vi "HFRR ADV v019 new software.vi"() -> ()   [LabVIEW 2025] (continued)
                        n2544 = disable-structure shown="Disabled" {
                          frame Disabled {
                            n2545 = local read "EVENT LOG"() -> (w3561:string)
                            n2546 = call "Event Log.vi"("Content"="Test Parameter", "EVENT LOG"=w3561) -> ("EVENT LOG"=w3560:string)  [unwired: 8 in, 1 out]
                            n2547 = local write "EVENT LOG"(w3560) -> ()
                          }
                          frame Enabled {
                          }
                        }
                      }
                      frame #20 {
                        n2548 = Wait (ms)(milliseconds to wait=u32 50) -> ()  [unwired: 1 out]
                      }
                      frame #21 {
                        n2549 = local read "Set Hz"() -> (w3565:dbl)
                        n2550 = Number To Fractional String(number=w3565, precision (6)=i16 2) -> (F-format string=w3564:string)  [unwired: 2 in]
                        n2551 = Concatenate Strings("Set Frequency [Hz] :" ("Content"), w3564) -> (w3567:string)
                        n2552 = local read "EVENT LOG"() -> (w3569:string)
                        n2553 = call "Event Log.vi"("Content"=w3567, "EVENT LOG"=w3569) -> ("EVENT LOG"=w3568:string)  [unwired: 8 in, 1 out]
                        n2554 = local write "EVENT LOG"(w3568) -> ()
                      }
                      frame #22 {
                        n2555 = Wait (ms)(milliseconds to wait=u32 50) -> ()  [unwired: 1 out]
                      }
                      frame #23 {
                        n2556 = local read "NORMAL LOAD"() -> (w3572:dbl)
                        n2557 = Number To Fractional String(number=w3572, precision (6)=i16 2) -> (F-format string=w3573:string)  [unwired: 2 in]
                        n2558 = Concatenate Strings("Applied Load [grams] :" ("Content"), w3573) -> (w3575:string)
                        n2559 = local read "EVENT LOG"() -> (w3577:string)
                        n2560 = call "Event Log.vi"("Content"=w3575, "EVENT LOG"=w3577) -> ("EVENT LOG"=w3576:string)  [unwired: 8 in, 1 out]
                        n2561 = local write "EVENT LOG"(w3576) -> ()
                      }
                      frame #24 {
                        n2562 = Wait (ms)(milliseconds to wait=u32 50) -> ()  [unwired: 1 out]
                      }
                      frame #25 {
                        n2563 = local read "Set Strk"() -> (w3580:dbl)
                        n2564 = Number To Fractional String(number=w3580, precision (6)=i16 2) -> (F-format string=w3581:string)  [unwired: 2 in]
                        n2565 = Concatenate Strings("Set Stroke [mm] :" ("Content"), w3581) -> (w3583:string)
                        n2566 = local read "EVENT LOG"() -> (w3585:string)
                        n2567 = call "Event Log.vi"("Content"=w3583, "EVENT LOG"=w3585) -> ("EVENT LOG"=w3584:string)  [unwired: 8 in, 1 out]
                        n2568 = local write "EVENT LOG"(w3584) -> ()
                      }
                      frame #26 {
                        n2569 = Wait (ms)(milliseconds to wait=u32 50) -> ()  [unwired: 1 out]
                      }
                      frame #27 {
                        n2570 = local read "Set Temp"() -> (w3588:dbl)
                        n2571 = Number To Fractional String(number=w3588, precision (6)=i16 2) -> (F-format string=w3589:string)  [unwired: 2 in]
                        n2572 = Concatenate Strings("Set Temperature [deg C] :" ("Content"), w3589) -> (w3591:string)
                        n2573 = local read "EVENT LOG"() -> (w3593:string)
                        n2574 = call "Event Log.vi"("Content"=w3591, "EVENT LOG"=w3593) -> ("EVENT LOG"=w3592:string)  [unwired: 8 in, 1 out]
                        n2575 = local write "EVENT LOG"(w3592) -> ()
                      }
                      frame #28 {
                        n2576 = Wait (ms)(milliseconds to wait=u32 50) -> ()  [unwired: 1 out]
                      }
                      frame #29 {
                        n2577 = local read "Set Rh"() -> (w3596:dbl)
                        n2578 = Number To Fractional String(number=w3596, precision (6)=i16 2) -> (F-format string=w3597:string)  [unwired: 2 in]
                        n2579 = Concatenate Strings("Set Humidity [%RH] :" ("Content"), w3597) -> (w3599:string)
                        n2580 = local read "EVENT LOG"() -> (w3601:string)
                        n2581 = call "Event Log.vi"("Content"=w3599, "EVENT LOG"=w3601) -> ("EVENT LOG"=w3600:string)  [unwired: 8 in, 1 out]
                        n2582 = local write "EVENT LOG"(w3600) -> ()
                      }
                      frame #30 {
                        n2583 = Wait (ms)(milliseconds to wait=u32 50) -> ()  [unwired: 1 out]
                      }
                      frame #31 {
                        n2584 = local read "test time"() -> (w3604:dbl)
                        n2585 = Number To Fractional String(number=w3604, precision (6)=i16 1) -> (F-format string=w3605:string)  [unwired: 2 in]
                        n2586 = Concatenate Strings("Test Duration [mins] :" ("Content"), w3605) -> (w3607:string)
                        n2587 = local read "EVENT LOG"() -> (w3609:string)
                        n2588 = call "Event Log.vi"("Content"=w3607, "EVENT LOG"=w3609) -> ("EVENT LOG"=w3608:string)  [unwired: 8 in, 1 out]
                        n2589 = local write "EVENT LOG"(w3608) -> ()
                      }
                      frame #32 {
                        w3610 = dbl[] [] ("History Data")
                        w3611 = cluster{"y":dbl, dbl, "y":dbl}[] [] ("History Data")
                        w3612 = FALSE ("Visible")
                        n2590 = property on="Stroke ( mm )" class="WFChart (strict)"("History Data"=w3611) -> ()  [unwired: 2 in, 2 out]
                        n2591 = property on="Humidity ( %RH )" class="WFChart (strict)"("History Data"=w3610) -> ()  [unwired: 2 in, 2 out]
                        n2592 = property on="Temperature ( Deg C )" class="WFChart (strict)"("History Data"=w3610) -> ()  [unwired: 2 in, 2 out]
                        n2593 = property on="Electrical Contact Resistance ( % )" class="WFChart (strict)"("History Data"=w3610) -> ()  [unwired: 2 in, 2 out]
                        n2594 = property on="Coefficient of Friction" class="WFChart (strict)"("History Data"=w3610) -> ()  [unwired: 2 in, 2 out]
                        n2595 = property on="Frictional Force ( N )" class="WFChart (strict)"("History Data"=w3610) -> ()  [unwired: 2 in, 2 out]
                        n2596 = property on="Coefficient of Friction" class="WFChart (strict)"("History Data"=w3610) -> ()  [unwired: 2 in, 2 out]
                        n2597 = property on="Frictional Force ( N )" class="WFChart (strict)"("History Data"=w3610) -> ()  [unwired: 2 in, 2 out]
                        n2598 = property on="Electrical Contact Resistance ( % )" class="WFChart (strict)"("History Data"=w3610) -> ()  [unwired: 2 in, 2 out]
                        n2599 = property on="Humidity ( %RH )" class="WFChart (strict)"("History Data"=w3610) -> ()  [unwired: 2 in, 2 out]
                        n2600 = property on="Stroke ( mm )" class="WFChart (strict)"("History Data"=w3611) -> ()  [unwired: 2 in, 2 out]
                        n2601 = property on="Temperature ( Deg C )" class="WFChart (strict)"("History Data"=w3610) -> ()  [unwired: 2 in, 2 out]
                        n2602 = property on="Service Password Log" class="Str"("Visible"=w3612) -> ()  [unwired: 2 in, 2 out]
                        n2603 = property on="Password 3" class="Clust (strict)"("Visible"=w3612) -> ()  [unwired: 2 in, 2 out]
                      }
                    }
                    "TEST FILE NAM,E SAVED" <- TRUE ("TEST FILE NAM,E SAVED")
                  }
                }
              }
            }
          }
        }
        n2604 = case shown="True" w2909 {
          frame False {
            n2605 = local write "tfalg"(0.0 ("tfalg")) -> ()
          }
          frame True {
            n2606 = local read "tfalg"() -> (w3054:dbl)
            n2607 = Equal?(x=w3054, y=0.0) -> (x = y?=w3055:bool)
            n2608 = case shown="True" w3055 {
              frame False {
              }
              frame True {
                n2609 = local read "Total No. of Tests"() -> (w3058:dbl)
                n2610 = local write "tfalg"(1.0 ("tfalg")) -> ()
                n2611 = local write "acq 2"(FALSE ("acq 2")) -> ()
                n2612 = Wait (ms)(milliseconds to wait=u32 200) -> ()  [unwired: 1 out]
                n2613 = Increment(x=w3058) -> (x+1=w3057:dbl)
                n2614 = local write "Total No. of Tests"(w3057) -> ()
              }
            }
          }
        }
        n2615 = local write "Test \nStatus"(w2915) -> ()
        n2616 = local write "Save"(w2915) -> ()
        n2617 = local read "Main Tab"() -> (w2872:T2)
        n2618 = case shown="True" w2896 {
          tunnel: [FALSE ("RUN") TRUE ("RUN")] -> w2895
          tunnel: [_ 1] -> w2888
          frame False {
          }
          frame True {
          }
        }
        n2619 = In Range and Coerce(upper limit=w2903, x=w2876, lower limit=w2902) -> (In Range?=w2894:bool)  [unwired: 1 out]
        n2620 = In Range and Coerce(upper limit=w2900, x=w2875, lower limit=w2901) -> (In Range?=w2892:bool)  [unwired: 1 out]
        n2621 = case shown="True" w2908 {
          frame False {
            n2622 = local read "Rt 3"() -> (w3036:bool)
            n2623 = case shown="True" w3036 {
              frame False {
              }
              frame True {
                n2624 = local write "Rt 3"(FALSE ("Rt 3")) -> ()
                n2625 = local write "Json End Flg"(TRUE ("Upld AR 2")) -> ()
              }
            }
            "Rt" <- TRUE ("Rt")
            "Rt 2" <- FALSE ("Rt")
          }
          frame True {
            n2626 = local read "Rt"() -> (w3043:bool)
            n2627 = local write "Rt 2"(TRUE ("Rt 2")) -> ()
            n2628 = case shown="True" w3043 {
              frame False {
              }
              frame True {
                w3044 = TRUE ("Upld AR 2")
                n2629 = local write "Rt"(FALSE ("Rt")) -> ()
                n2630 = local write "Upld AR"(w3044) -> ()
                n2631 = local write "Json St Flg"(w3044) -> ()
              }
            }
            "Rt 3" <- TRUE ("Rt 3")
          }
        }
        n2632 = case shown="True" w2894 {
          tunnel: [FALSE ("RUN") TRUE ("RUN")] -> w2893
          tunnel: [_ 2] -> w2887
          frame False {
          }
          frame True {
          }
        }
        n2633 = case shown="True" w2892 {
          tunnel: [FALSE ("RUN") TRUE ("RUN")] -> w2891
          tunnel: [_ 3] -> w2886
          frame False {
          }
          frame True {
          }
        }
        n2634 = case shown="\"Acquire\"" w2872 {
          tunnel: w2874 -> [_ w3105]
          frame Default {
            w3104 = 0.0 ("output")
            n2635 = local write "PID-out"(w3104) -> ()
            n2636 = local write "Frequency ( Hz )"(w3104) -> ()
          }
          frame "Acquire" {
            n2637 = stacked-sequence {
              frame #0 {
                n2638 = local read "Auto Start Test"() -> (w3107:bool)
                n2639 = case shown="True" w3107 {
                  tunnel: "RUN" -> [w3128 w3131]
                  tunnel: [w3128 w3130] -> w3108
                  frame False {
                  }
                  frame True {
                    n2640 = local read "Auto Start Temp"() -> (w3129:bool)
                    n2641 = Or(x=w3131, y=w3129) -> (x .or. y?=w3130:bool)
                  }
                }
                n2642 = local read "clk"() -> (w3127:dbl)
                n2643 = local read "Save"() -> (w3123:bool)
                n2644 = Equal?(x=w3127, y=0.0) -> (x = y?=w3124:bool)
                n2645 = And(x=w3124, y=w3123) -> (x .and. y?=w3125:bool)
                n2646 = Not(x="Engage") -> (.not. x?=w3114:bool)
                n2647 = case shown="False" w3108 {
                  tunnel: [0.0 w3154] -> w3110
                  frame False {
                    (unwired) TRUE ("Visible")
                    n2648 = local read "Auto Start Test"() -> (w3135:bool)
                    n2649 = local write "Start Time"(TRUE ("Start Time")) -> ()
                    n2650 = property on="Stroke 2" class="DigNum (strict)"("Visible"=FALSE) -> ()  [unwired: 2 in, 2 out]
                    n2651 = case shown="False" w3135 {
                      frame False {
                        n2652 = property on="Heater Button" class="Bool (strict)"("DisabledEnum"=T19."Enabled" ("Disabled")) -> ()  [unwired: 2 in, 2 out]
                        n2653 = property on="Humidity" class="Bool (strict)"("DisabledEnum"=T19."Enabled" ("Disabled")) -> ()  [unwired: 2 in, 2 out]
                      }
                      frame True {
                      }
                    }
                    n2654 = case shown="False" "TestCompFlg" {
                      frame False {
                        n2655 = local read "StartFlg"() -> (w3143:bool)
                        n2656 = case shown="True" w3143 {
                          frame False {
                          }
                          frame True {
                            n2657 = stacked-sequence {
                              frame #0 {
                                n2658 = local read "EVENT LOG"() -> (w3147:string)
                                n2659 = call "Event Log.vi"("Content"="Test was interrupted", "EVENT LOG"=w3147) -> ("EVENT LOG"=w3148:string)  [unwired: 8 in, 1 out]
                                n2660 = local write "EVENT LOG"(w3148) -> ()
                                n2661 = property on="RUN" class="Bool (strict)"("Visible"=TRUE) -> ()  [unwired: 2 in, 2 out]
                                n2662 = property on="Auto Start Test" class="Bool (strict)"("Visible"=TRUE) -> ()  [unwired: 2 in, 2 out]
                              }
                              frame #1 {
                                w3150 = FALSE ("StartFlg")
                                n2663 = property on="Heater Button" class="Bool (strict)"("Val(Sgnl)"=FALSE ("Value (Signaling)")) -> ()  [unwired: 2 in, 2 out]
                                n2664 = local write "Heater Button"(w3150) -> ()
                                n2665 = local write "StartFlg"(w3150) -> ()
                                n2666 = local write "Humidity"(w3150) -> ()
                              }
                              frame #2 {
                                n2667 = local write "Command"("VC;0" ("Command")) -> ()
                              }
                              frame #3 {
                                n2668 = Wait (ms)(milliseconds to wait=u32 1500) -> ()  [unwired: 1 out]
                              }
                              frame #4 {
                                n2669 = local write "Command"("HE;0" ("Command")) -> ()
                              }
                            }
                          }
                        }
                      }
                      frame True {
                      }
                    }
                    n2670 = local write "String 14"("Test will autostart once parameters reach the set value." ("String 14")) -> ()
                  }
                  frame True {
                    (unwired) FALSE ("Visible")
                    n2671 = property on="Stroke 2" class="DigNum (strict)"("Visible"=TRUE) -> ()  [unwired: 2 in, 2 out]
                    n2672 = property on="STOP 2" class="Bool (strict)"("Disabled"=u8 2) -> ()  [unwired: 2 in, 2 out]
                    n2673 = local write "String 14"(" Running....." ("String 14")) -> ()
                    n2674 = property on="Heater Button" class="Bool (strict)"("DisabledEnum"=T19."Disabled and Grayed Out" ("Disabled")) -> ()  [unwired: 2 in, 2 out]
                    n2675 = property on="Humidity" class="Bool (strict)"("DisabledEnum"=T19."Disabled and Grayed Out" ("Disabled")) -> ()  [unwired: 2 in, 2 out]
                    n2676 = case shown="True" "Start Time" {
                      selector: "Start Time" -> [_ w3173]
                      frame False {
                      }
                      frame True {
                        n2677 = Not(x=w3173) -> (.not. x?=w3172:bool)
                        n2678 = local write "Start Time"(w3172) -> ()
                        n2679 = local read "EVENT LOG"() -> (w3174:string)
                        n2680 = call "Event Log.vi"("Content"="Test in progress", "EVENT LOG"=w3174) -> ("EVENT LOG"=w3176:string)  [unwired: 8 in, 1 out]
                        n2681 = local write "EVENT LOG"(w3176) -> ()
                      }
                    }
                    n2682 = disable-structure shown="Enabled" {
                      disable-tunnel: [w3165 w3171] -> w3154
                      frame Disabled {
                        n2683 = local read "Set Hz"() -> (w3168:dbl)
                        n2684 = call <vilib>:"Uniform White Noise Waveform.vi"() -> ("signal out"=w3167:waveform(dbl))  [unwired: 10 in, 1 out]
                        n2685 = Random Number (0-1)() -> (number: 0 to 1=w3164:dbl)
                        n2686 = Add(x=w3168, y=w3167) -> (x+y=w3166:waveform(dbl))
                        n2687 = Multiply(x=ext 0.01 ("y"), y=w3164) -> (x*y=w3162:ext)
                        n2688 = Multiply(x=w3166, y=w3162) -> (x*y=w3165:waveform(ext))
                      }
                      frame Enabled {
                        n2689 = call-poly <vilib>:"Random Number (Range).vi"("lower bound (0)"=49.89, "upper bound (100)"=50.8) -> ("number"=w3171:dbl)  [unwired: 9 in]
                      }
                    }
                    "StartFlg" <- TRUE ("StartFlg")
                  }
                }
                n2690 = case shown="True" w3125 {
                  frame False {
                  }
                  frame True {
                    n2691 = local write "clk"(10.0 ("clk")) -> ()
                    n2692 = Get Date/Time In Seconds() -> (seconds since 1Jan1904=w3179:timestamp)
                    n2693 = To Double Precision Float(number=w3179) -> (double precision float=w3177:dbl)
                    n2694 = local write "acq timer"(w3177) -> ()
                    n2695 = local write "act save time"(w3177) -> ()
                  }
                }
                n2696 = call "Elapsed Time"("Time Target (s)"="Countdown", "Reset"=w3114) -> ("Elapsed Time (s)"=w3119:dbl, "Time has Elapsed"=w3117:bool)  [unwired: 10 in, 6 out]
                "Countdown 2" <- w3119
                n2697 = Subtract(x=w3119, y=2.0) -> (x-y=w3122:dbl)
                n2698 = Less?(x=w3122, y="Countdown") -> (x < y?=w3120:bool)
                n2699 = And(x=w3120, y=w3117) -> (x .and. y?=w3116:bool)
                n2700 = case shown="True" w3116 {
                  frame False {
                  }
                  frame True {
                    (unwired) dbl[] [] ("History Data")
                    n2701 = local write "Engage"(FALSE ("Engage")) -> ()
                    n2702 = local write "RUN"(TRUE ("RUN")) -> ()
                    n2703 = local read "Humidity ( %RH )"() -> (→"Rh Before":dbl)
                  }
                }
                n2704 = local read "Test \nStatus"() -> (w3112:bool)
                n2705 = Select(t=w3110, s=w3112, f=0.0) -> (s? t:f=w3111:dbl)
                n2706 = local write "Frequency ( Hz )"(w3111) -> ()
              }
              frame #1 {
                w3202 = 1000000.0 ("x")
                # "HC;1/0\nST;VALUE"
                # "Elapsed time\ncof\nstroke\nAir temp\nTemp\nHumidity"
                # "acq timer\n\nact save time"
                # "convert to microseconds"
                n2707 = local read "COUNT"() -> (w3185:i32)
                n2708 = local read "Rate"() -> (w3198:dbl)
                n2709 = Divide(x=w3202, y=w3198) -> (x/y=w3203:dbl)
                n2710 = Greater Or Equal?(x=w3185, y=250) -> (x >= y?=w3184:bool)
                n2711 = Get Date/Time In Seconds() -> (seconds since 1Jan1904=w3205:timestamp)
                n2712 = case shown="True" w3184 {
                  frame False {
                    n2713 = local read "COUNT"() -> (w3206:i32)
                    n2714 = Increment(x=w3206) -> (x+1=w3207:i32)
                    n2715 = local write "COUNT"(w3207) -> ()
                  }
                  frame True {
                    n2716 = local write "COUNT"(0 ("COUNT")) -> ()
                  }
                }
                n2717 = local read "Samplingtime 2"() -> (w3183:dbl)
                n2718 = local read "act save time"() -> (w3200:dbl)
                n2719 = Divide(x=w3203, y=w3202) -> (x/y=w3201:dbl)
                n2720 = To Double Precision Float(number=w3205) -> (double precision float=w3194:dbl)
                n2721 = Add(x=w3200, y=w3183) -> (x+y=w3199:dbl)
                n2722 = local read "acq timer"() -> (w3204:dbl)
                n2723 = local read "COUNT"() -> (w3187:i32)
                n2724 = Greater Or Equal?(x=w3194, y=w3199) -> (x >= y?=w3182:bool)
                n2725 = Multiply(x=w3201, y=w3187) -> (x*y=w3193:dbl)
                n2726 = Subtract(x=w3194, y=w3204) -> (x-y=w3196:dbl)
                n2727 = local read "Save"() -> (w3197:bool)
                n2728 = Add(x=w3196, y=w3193) -> (x+y=w3180:dbl)
                "Elapsed time 3" <- w3180
                n2729 = And(x=w3182, y=w3197) -> (x .and. y?=w3195:bool)
                n2730 = Divide(x=w3180, y=60.0) -> (x/y=w3191:dbl)
                n2731 = local read "Test \nStatus"() -> (w3181:bool)
                n2732 = local read "clk"() -> (w3188:dbl)
                n2733 = Equal?(x=w3188, y=10.0) -> (x = y?=w3190:bool)
                n2734 = case shown="True" w3195 {
                  tunnel: w3194 -> [_ w3318]
                  tunnel: [FALSE ("Boolean 2") TRUE ("Boolean 2")] -> _
                  frame False {
                  }
                  frame True {
                    w3272 = ";" ("Substring")
                    # "Pid out/\nFreq response value"
                    n2735 = local write "act save time"(w3318) -> ()
                    n2736 = local read "FILE"() -> (w3266:string)
                    n2737 = call "file check.vi"("file name in"=w3266) -> ("error out"=w3269:errorcluster, "file name out"=w3264:string)  [unwired: 9 in]
                    n2738 = local read "LVDT STROKE"() -> (w3261:dbl)
                    n2739 = local read "Add up Stroke"() -> (w3259:dbl)
                    n2740 = call "FILE PATH CREATION.vi"("error in"=w3269, "FILE NAME :"=w3264) -> ("FILE OUT"=w3267:path)  [unwired: 8 in, 1 out]
                    n2741 = Concatenate Strings(w3264, ".dgf" ("Substring")) -> (w3268:string)
                    n2742 = Subtract(x=w3261, y=w3259) -> (x-y=w3260:dbl)
                    n2743 = Absolute Value(x=w3260) -> (abs(x)=w3258:dbl)
                    n2744 = local read "FF 2"() -> (→"Frictional Force ( N )" →"Frictional Force ( N )":dbl)
                    n2745 = Build Path(base path=w3267, name or relative path=w3268) -> (appended path=w3263:path)
                    n2746 = local read "COF 2"() -> (w3277:dbl)
                    "cof" <- w3277
                    "Coefficient of Friction" <- w3277
                    "COF 4" <- w3277
                    "Coefficient of Friction" <- w3277
                    n2747 = local read "TEMP"() -> (w3280:dbl)
                    "Temp" <- w3280
                    "Temperature ( Deg C )" <- w3280
                    n2748 = local read "Humidity ( %RH )"() -> (w3279:dbl)
                    "Humidity ( %RH )" <- w3279
                    "Humidity ( %RH )" <- w3279
                    n2749 = local read "Frequency ( Hz )"() -> (w3286:dbl)
                    n2750 = call <vilib>:"Mean PtByPt.vi"("x"=w3258, "sample length"="STROKE FILTER") -> ("mean"=w3257:dbl)  [unwired: 2 in, 1 out]
                    n2751 = local read "Elapsed time"() -> (w3311:dbl)
                    n2752 = local read "AIR TEMP"() -> (w3284:dbl)
                    n2753 = local read "PID-out"() -> (w3289:dbl)
                    n2754 = local write "Temperature ( Deg C )"(w3280) -> ()
                    n2755 = Number To Fractional String(number=w3257, width (-)=i16 9 ("precision (6)"), precision (6)=i16 6) -> (F-format string=w3304:string)  [unwired: 1 in]
                    n2756 = Number To Fractional String(number=w3284, width (-)=i16 9 ("precision (6)"), precision (6)=i16 3) -> (F-format string=w3303:string)  [unwired: 1 in]
                    n2757 = Number To Fractional String(number=w3280, width (-)=i16 9 ("precision (6)"), precision (6)=i16 3) -> (F-format string=w3300:string)  [unwired: 1 in]
                    n2758 = Number To Fractional String(number=w3279, width (-)=i16 9 ("precision (6)"), precision (6)=i16 3) -> (F-format string=w3297:string)  [unwired: 1 in]
                    n2759 = Number To Fractional String(number=0.0, width (-)=i16 9 ("precision (6)"), precision (6)=i16 3) -> (F-format string=w3294:string)  [unwired: 1 in]
                    n2760 = Number To Fractional String(number=w3289, width (-)=i16 9 ("precision (6)"), precision (6)=i16 3) -> (F-format string=w3290:string)  [unwired: 1 in]
                    n2761 = Number To Fractional String(number=w3286, width (-)=i16 9 ("precision (6)"), precision (6)=i16 3) -> (F-format string=w3285:string)  [unwired: 1 in]
                    n2762 = Number To Fractional String(number=w3277, width (-)=i16 9 ("precision (6)"), precision (6)=i16 6) -> (F-format string=w3312:string)  [unwired: 1 in]
                    n2763 = Number To Fractional String(number=w3311, width (-)=i16 14 ("precision (6)"), precision (6)=i16 3) -> (F-format string=w3313:string)  [unwired: 1 in]
                    n2764 = Bundle("y"=1.02, "mean"=w3257, "y"=0.98) -> (w3278:cluster{"y":dbl, "mean":dbl, "y":dbl})  [unwired: 1 in]
                    n2765 = Number To Fractional String(number="Ambient Humidity :", width (-)=i16 9 ("precision (6)"), precision (6)=i16 6) -> (F-format string=w3270:string)  [unwired: 1 in]
                    n2766 = local read "RUN"() -> (w3276:bool)
                    n2767 = case shown="True" w3276 {
                      tunnel: w3278 -> [_ w3323]
                      tunnel: w3257 -> [_ w3322]
                      tunnel: w3257 -> [_ w3320]
                      tunnel: w3257 -> [_ w3321]
                      frame False {
                      }
                      frame True {
                        "Stroke ( mm )" <- w3323
                        "Stroke ( mm )" <- w3323
                        "Stroke 4" <- w3322
                        "Stroke 3" <- w3320
                        "Stroke 2" <- w3321
                        "measured_stroke" <- w3320
                      }
                    }
                    n2768 = Concatenate Strings(w3313, w3272, w3312, w3272, w3304, w3272, w3303, w3272, w3300, w3272, w3297, w3272, w3294, w3272, w3290, w3272, w3285, w3272, w3270, "\r") -> (w3310:string)
                    n2769 = call <vilib>:"Write Characters To File.vi"("append to file? (new file:F)"=TRUE, "character string"=w3310, "file path (dialog if empty)"=w3263) -> ()  [unwired: 2 in, 1 out]
                    "refresh flag" <- TRUE ("refresh flag")
                  }
                }
                n2770 = case shown="True" w3181 {
                  tunnel: w3191 -> [_ w3217]
                  tunnel: w3196 -> [_ w3227]
                  tunnel: [0.0 w3223] -> _
                  tunnel: w3190 -> [_ w3222]
                  tunnel: [0.0 w3221] -> _
                  tunnel: w3180 -> [_ w3221]
                  tunnel: w3194 -> [w3210 _]
                  frame False {
                    n2771 = local write "acq timer"(w3210) -> ()
                    n2772 = local write "Test Duration Status"(0.0 ("Test Duration Status")) -> ()
                  }
                  frame True {
                    n2773 = local read "Set Hz"() -> (w3224:dbl)
                    n2774 = local write "Elapsed time"(w3217) -> ()
                    n2775 = local read "test time"() -> (w3216:dbl)
                    n2776 = Multiply(x=w3227, y=w3224) -> (x*y=w3226:dbl)
                    n2777 = case shown="False" w3222 {
                      tunnel: w3226 -> [w3228 _]
                      tunnel: [w3228 1.0] -> w3223
                      frame False {
                        n2778 = local write "Cycles elapsed"(w3228) -> ()
                      }
                      frame True {
                      }
                    }
                    n2779 = Greater?(x=w3217, y=w3216) -> (0:w3225:bool)
                    n2780 = Subtract(x=w3216, y=w3217) -> (x-y=w3215:dbl)
                    "time" <- w3215
                    n2781 = Multiply(x=w3215, y=60.0) -> (x*y=w3214:dbl)
                    n2782 = local write "Time Remaining"(w3214) -> ()
                    n2783 = local write "Remaining Time"(w3214) -> ()
                    n2784 = case shown="True" w3225 {
                      frame False {
                      }
                      frame True {
                        n2785 = stacked-sequence {
                          frame #0 {
                            w3233 = T19."Enabled" ("Disabled")
                            w3232 = FALSE ("TEST FILE NAM,E SAVED")
                            w3234 = "" ("FILE")
                            w3235 = TRUE ("Visible")
                            n2786 = local write "Humidity"(FALSE ("Humidity")) -> ()
                            n2787 = local write "RUN"(FALSE ("OK Button 2")) -> ()
                            n2788 = local write "Heater Button"(FALSE ("Heater Button")) -> ()
                            n2789 = local write "Auto Start Test"(FALSE ("Auto Start Test")) -> ()
                            n2790 = local write "TestCompFlg"(TRUE ("StpFlg")) -> ()
                            n2791 = local read "Humidity ( %RH )"() -> (→"Rh After":dbl)
                            n2792 = property on="STOP 2" class="Bool (strict)"("Disabled"=u8 0) -> ()  [unwired: 2 in, 2 out]
                            n2793 = local read "EVENT LOG"() -> (w3240:string)
                            n2794 = call "Event Log.vi"("Content"="Test Completed", "EVENT LOG"=w3240) -> ("EVENT LOG"=w3239:string)  [unwired: 8 in, 1 out]
                            n2795 = property on="RUN" class="Bool (strict)"("Visible"=w3235) -> ()  [unwired: 2 in, 2 out]
                            n2796 = property on="Auto Start Test" class="Bool (strict)"("Visible"=w3235) -> ()  [unwired: 2 in, 2 out]
                            n2797 = local write "Batch Ref Num :"(w3234) -> ()
                            n2798 = local write "FILE"(w3234) -> ()
                            n2799 = local write "EVENT LOG"(w3239) -> ()
                            n2800 = local write "TEST FILE NAM,E SAVED"(w3232) -> ()
                            n2801 = local write "Fuel Discription :"(w3234) -> ()
                            n2802 = local write "START TEMP"(w3232) -> ()
                            n2803 = local write "Remarks :"(w3234) -> ()
                            n2804 = local write "Main Dashboard Buttons"(T1."Imaging" ("Main Dashboard Buttons")) -> ()
                            n2805 = local write "Main Tab"(T2."Adv Scar" ("Main Tab")) -> ()
                            n2806 = property on="FRICVALZ 2" class="Bool (strict)"("DisabledEnum"=w3233) -> ()  [unwired: 2 in, 2 out]
                            n2807 = property on="FRICVALZ 3" class="Bool (strict)"("DisabledEnum"=w3233) -> ()  [unwired: 2 in, 2 out]
                            n2808 = property on="FRICVALZ 4" class="Bool (strict)"("DisabledEnum"=w3233) -> ()  [unwired: 2 in, 2 out]
                          }
                          frame #1 {
                            n2809 = Wait (ms)(milliseconds to wait=u32 1500) -> ()  [unwired: 1 out]
                          }
                          frame #2 {
                            n2810 = local write "Command"("VC;0") -> ()
                          }
                          frame #3 {
                            n2811 = Wait (ms)(milliseconds to wait=u32 1500) -> ()  [unwired: 1 out]
                          }
                          frame #4 {
                            n2812 = local write "Command"("VC;0") -> ()
                          }
                          frame #5 {
                            n2813 = Wait (ms)(milliseconds to wait=u32 1500) -> ()  [unwired: 1 out]
                          }
                          frame #6 {
                            n2814 = local write "Command"("ST;0") -> ()
                          }
                          frame #7 {
                            n2815 = local write "measured_stroke"(0.0 ("measured_stroke")) -> ()
                            n2816 = Wait (ms)(milliseconds to wait=u32 1500) -> ()  [unwired: 1 out]
                          }
                          frame #8 {
                            n2817 = local write "Command"("HE;0") -> ()
                          }
                        }
                      }
                    }
                    n2818 = Divide(x=w3217, y=w3216) -> (x/y=w3220:dbl)
                    n2819 = Multiply(x=w3220, y=100.0) -> (x*y=w3218:dbl)
                    n2820 = local write "Test Duration Status"(w3218) -> ()
                  }
                }
              }
              frame #2 {
                n2821 = case shown="True" "Heater Button" {
                  tunnel: [0.0 ("output") w3346] -> w3324
                  frame False {
                    w3327 = TRUE ("tmpchk")
                    n2822 = local read "TEMP"() -> (w3328:dbl)
                    n2823 = local write "Temp ini"(w3328) -> ()
                    n2824 = local write "Reset 4"(w3327) -> ()
                    n2825 = local write "tmpchk"(w3327) -> ()
                    n2826 = local write "reinit"(TRUE ("reinit")) -> ()
                    n2827 = local write "manual temp log"(TRUE ("manual temp log")) -> ()
                  }
                  frame True {
                    # "Logic to turn off\nthe heater when \ntemp is not rising.\nTime - 60 sec\nDelta t- 5°c"
                    n2828 = local read "Temp ini"() -> (w3335:dbl)
                    n2829 = local read "Auto Start Test"() -> (w3331:bool)
                    n2830 = Less?(x=w3335, y=53.0) -> (x < y?=w3333:bool)
                    n2831 = case shown="False" w3331 {
                      frame False {
                        n2832 = local read "Set Temp"() -> (w3355:dbl)
                        n2833 = local read "TEMP"() -> (w3354:dbl)
                        n2834 = Subtract(x=w3355, y=w3354) -> (x-y=w3353:dbl)
                        n2835 = Absolute Value(x=w3353) -> (abs(x)=w3352:dbl)
                        n2836 = Less?(x=w3352, y=0.5) -> (x < y?=w3350:bool)
                        n2837 = case shown="True" w3350 {
                          tunnel: "manual temp log" -> [_ w3356]
                          frame False {
                          }
                          frame True {
                            n2838 = case shown="True" w3356 {
                              selector: w3356 -> [_ w3357]
                              frame False {
                              }
                              frame True {
                                # "#Event log"
                                n2839 = Not(x=w3357) -> (.not. x?=w3358:bool)
                                n2840 = local write "manual temp log"(w3358) -> ()
                                n2841 = local read "EVENT LOG"() -> (w3361:string)
                                n2842 = call "Event Log.vi"("Content"="Target Temperature reached", "EVENT LOG"=w3361) -> ("EVENT LOG"=w3360:string)  [unwired: 8 in, 1 out]
                                n2843 = local write "EVENT LOG"(w3360) -> ()
                              }
                            }
                          }
                        }
                      }
                      frame True {
                        n2844 = local write "manual temp log"(TRUE ("manual temp log")) -> ()
                      }
                    }
                    n2845 = And(x="tmpchk", y=w3333) -> (x .and. y?=w3336:bool)
                    n2846 = case shown="True" w3336 {
                      frame False {
                      }
                      frame True {
                        n2847 = call "Elapsed Time8"("Time Target (s)"=300.0, "Reset"="Reset 4") -> ("Time has Elapsed"=w3363:bool)  [unwired: 10 in, 7 out]
                        n2848 = flat-sequence {
                          tunnel: w3363 -> [_]
                          frame #0 {
                            n2849 = local write "Reset 4"(FALSE ("Reset 4")) -> ()
                          }
                        }
                        n2850 = case shown="True" w3363 {
                          frame False {
                          }
                          frame True {
                            n2851 = local read "Temp ini"() -> (w3370:dbl)
                            n2852 = Add(x=w3370, y=5.0) -> (x+y=w3368:dbl)
                            n2853 = local read "TEMP"() -> (w3371:dbl)
                            n2854 = Greater?(x=w3371, y=w3368) -> (0:w3369:bool)
                            n2855 = case shown="False" w3369 {
                              frame False {
                                n2856 = local write "Heater Button"(FALSE ("Heater Button")) -> ()
                              }
                              frame True {
                                n2857 = local write "tmpchk"(FALSE ("tmpchk")) -> ()
                              }
                            }
                          }
                        }
                      }
                    }
                    n2858 = local read "Set Temp"() -> (w3344:dbl)
                    n2859 = local read "TEMP"() -> (w3338:dbl)
                    n2860 = call-poly <vilib>:"PID.vi"("reinitialize? (F)"="reinit", "dt (s)"=-1.0, "process variable"=w3338, "setpoint"=w3344) -> ("output"=w3341:dbl)  [unwired: 6 in, 1 out]
                    n2861 = Subtract(x=w3344, y=w3338) -> (x-y=w3345:dbl)
                    n2862 = Add(x=w3344, y=0.5) -> (x+y=w3342:dbl)
                    n2863 = Greater Or Equal?(x=w3338, y=w3342) -> ()  [unwired: 1 out]
                    n2864 = Select(t=0.0, s=FALSE, f=w3341) -> (s? t:f=w3340:dbl)
                    "PID output" <- w3340
                    n2865 = flat-sequence {
                      tunnel: w3340 -> [w3374]
                      tunnel: [w3374] -> w3346
                      frame #0 {
                        n2866 = local write "reinit"(FALSE ("reinit")) -> ()
                      }
                    }
                    n2867 = Bundle(w3345, "output"=w3340, "TEMP"=w3338) -> ()  [unwired: 1 in, 1 out]
                  }
                }
                "PID-out" <- w3324
              }
              frame #3 {
                n2868 = local read "TEMP"() -> (w3376:dbl)
                n2869 = Greater Or Equal?(x=w3376, y="Set Temp 2") -> (x >= y?=w3381:bool)
                n2870 = case shown="True" w3381 {
                  tunnel: [FALSE TRUE] -> w3379
                  frame False {
                  }
                  frame True {
                  }
                }
                "Status 13" <- w3379
                n2871 = And(x=w3379, y="trip1 8") -> (x .and. y?=w3378:bool)
                n2872 = case shown="True" w3378 {
                  frame False {
                    n2873 = local write "Heater Trip Temp"(TRUE ("Heater Trip Temp")) -> ()
                  }
                  frame True {
                    w3384 = FALSE ("OK Button 2")
                    n2874 = case shown="True" "Heater Trip Temp" {
                      selector: "Heater Trip Temp" -> [_ w3386]
                      frame False {
                      }
                      frame True {
                        n2875 = Not(x=w3386) -> (.not. x?=w3385:bool)
                        n2876 = local read "EVENT LOG"() -> (w3389:string)
                        n2877 = local write "Heater Trip Temp"(w3385) -> ()
                        n2878 = call "Event Log.vi"("Content"="Heater Trip", "EVENT LOG"=w3389) -> ("EVENT LOG"=w3388:string)  [unwired: 8 in, 1 out]
                        n2879 = local write "EVENT LOG"(w3388) -> ()
                      }
                    }
                    n2880 = local write "RUN"(w3384) -> ()
                    n2881 = property on="Auto Start Test" class="Bool (strict)"("Value"=w3384) -> ()  [unwired: 2 in, 2 out]
                    n2882 = local write "Heater Button"(w3384) -> ()
                  }
                }
              }
            }
            n2883 = case shown="False" w3105 {
              frame False {
                n2884 = disable-structure shown="Disabled" {
                  frame Disabled {
                    n2885 = stacked-sequence {
                      frame #0 {
                        n2886 = local write "RUN"(FALSE ("OK Button 2")) -> ()
                      }
                      frame #1 {
                      }
                    }
                  }
                  frame Enabled {
                  }
                }
              }
              frame True {
              }
            }
          }
        }
        n2887 = local read "airtempflg"() -> (w2897:bool)
        n2888 = Or(x=w2897, y=w2895) -> (x .or. y?=w2898:bool)
        n2889 = Insert Into Array(array=string[] ["Air Temperature has reached set value,", "Humidity has reached set value,", "Sample Temperaturehas reached set value,", ""], index=0, new element="") -> (w2883:string[])
        n2890 = Build Array(w2888, w2887, w2886) -> (w2884:i32[])
        n2891 = disable-structure shown="Disabled" {
          disable-tunnel: w2898 -> [w2975 _]
          disable-tunnel: w2893 -> [w2974 _]
          disable-tunnel: w2891 -> [w2973 _]
          frame Disabled {
            n2892 = Compound Arithmetic op=AND(w2975, w2974, w2973) -> ()  [unwired: 1 out]
            n2893 = case shown="True" {
              selector: _ -> [_ _]
              frame False {
              }
              frame True {
                w2976 = FALSE ("autostrtflg")
                n2894 = local write "RUN"(TRUE ("RUN")) -> ()
                n2895 = local write "autostrtflg"(w2976) -> ()
                n2896 = local write "autostart"(w2976) -> ()
                n2897 = local write "String 14"(" Running....." ("String 14")) -> ()
              }
            }
          }
          frame Enabled {
          }
        }
        n2898 = for {
          tunnel: w2884 -> [w3026] mode=indexing
          tunnel: w2883 -> [w3025]
          shift-right: [w3022] -> w2882
          shift-left: "" -> [w3024]
          n2899 = Index Array(array=w3025, index=w3026) -> (element=w3023:string)
          n2900 = Concatenate Strings(w3023, w3024) -> (w3022:string)
        }
        n2901 = local write "autostart 2"(w2882) -> ()
        n2902 = local read "Reset Graph"() -> (w2871:bool)
        n2903 = case shown="True" w2871 {
          selector: w2871 -> [_ w2925]
          frame False {
          }
          frame True {
            w2939 = 0.0 ("X Scale.Range:Maximum")
            n2904 = Not(x=w2925) -> (.not. x?=w2924:bool)
            n2905 = local write "Reset Graph"(w2924) -> ()
            n2906 = property on="Electrical Contact Resistance ( % )" class="WFChart (strict)"("XScale.Maximum"=600.0 ("X Scale.Range:Maximum"), "XScale.Minimum"=0.0 ("X Scale.Range:Minimum"), "YScale.Maximum"=100.0 ("Y Scale.Range:Maximum"), "YScale.Minimum"=0.0 ("Y Scale.Range:Minimum")) -> ()  [unwired: 2 in, 2 out]
            n2907 = property on="Frictional Force ( N )" class="WFChart (strict)"("XScale.Maximum"=600.0 ("X Scale.Range:Maximum"), "XScale.Minimum"=0.0 ("X Scale.Range:Minimum"), "YScale.Maximum"=100.0 ("Y Scale.Range:Maximum"), "YScale.Minimum"=0.0 ("Y Scale.Range:Minimum")) -> ()  [unwired: 2 in, 2 out]
            n2908 = property on="Temperature ( Deg C )" class="WFChart (strict)"("XScale.Maximum"=600.0 ("X Scale.Range:Maximum"), "XScale.Minimum"=0.0 ("X Scale.Range:Minimum"), "YScale.Maximum"=100.0 ("Y Scale.Range:Maximum"), "YScale.Minimum"=0.0 ("Y Scale.Range:Minimum")) -> ()  [unwired: 2 in, 2 out]
            n2909 = property on="Humidity ( %RH )" class="WFChart (strict)"("XScale.Maximum"=600.0 ("X Scale.Range:Maximum"), "XScale.Minimum"=0.0 ("X Scale.Range:Minimum"), "YScale.Maximum"=100.0 ("Y Scale.Range:Maximum"), "YScale.Minimum"=0.0 ("Y Scale.Range:Minimum")) -> ()  [unwired: 2 in, 2 out]
            n2910 = property on="Stroke ( mm )" class="WFChart (strict)"("XScale.Maximum"=600.0 ("X Scale.Range:Maximum"), "XScale.Minimum"=0.0 ("X Scale.Range:Minimum"), "YScale.Maximum"=100.0 ("Y Scale.Range:Maximum"), "YScale.Minimum"=0.0 ("Y Scale.Range:Minimum")) -> ()  [unwired: 2 in, 2 out]
            n2911 = property on="Coefficient of Friction" class="WFChart (strict)"("XScale.Maximum"=600.0 ("X Scale.Range:Maximum"), "XScale.Minimum"=0.0 ("X Scale.Range:Minimum"), "YScale.Maximum"=100.0 ("Y Scale.Range:Maximum"), "YScale.Minimum"=0.0 ("Y Scale.Range:Minimum")) -> ()  [unwired: 2 in, 2 out]
            n2912 = property on="Electrical Contact Resistance ( % )" class="WFChart (strict)"("XScale.Minimum"=0.0 ("X Scale.Range:Minimum"), "XScale.Maximum"=600.0 ("X Scale.Range:Maximum"), "YScale.Minimum"=0.0 ("Y Scale.Range:Minimum"), "YScale.Maximum"=100.0 ("Y Scale.Range:Maximum")) -> ()  [unwired: 2 in, 2 out]
            n2913 = property on="Temperature ( Deg C )" class="WFChart (strict)"("XScale.Minimum"=0.0 ("X Scale.Range:Minimum"), "XScale.Maximum"=600.0 ("X Scale.Range:Maximum"), "YScale.Minimum"=0.0 ("Y Scale.Range:Minimum"), "YScale.Maximum"=100.0 ("Y Scale.Range:Maximum")) -> ()  [unwired: 2 in, 2 out]
            n2914 = property on="Coefficient of Friction" class="WFChart (strict)"("XScale.Minimum"=0.0 ("X Scale.Range:Minimum"), "XScale.Maximum"=600.0 ("X Scale.Range:Maximum"), "YScale.Maximum"=1.0 ("X Scale.Range:Minimum"), "YScale.Minimum"=0.0 ("X Scale.Range:Minimum")) -> ()  [unwired: 2 in, 2 out]
            n2915 = property on="Frictional Force ( N )" class="WFChart (strict)"("XScale.Maximum"=600.0 ("X Scale.Range:Maximum"), "XScale.Minimum"=w2939, "YScale.Maximum"=10.0 ("Y Scale.Range:Maximum"), "YScale.Minimum"=w2939) -> ()  [unwired: 2 in, 2 out]
            n2916 = property on="Stroke ( mm )" class="WFChart (strict)"("XScale.Maximum"=600.0 ("X Scale.Range:Maximum"), "XScale.Minimum"=0.0 ("X Scale.Range:Minimum"), "YScale.Maximum"=100.0 ("Y Scale.Range:Maximum"), "YScale.Minimum"=0.0 ("Y Scale.Range:Minimum")) -> ()  [unwired: 2 in, 2 out]
            n2917 = property on="Humidity ( %RH )" class="WFChart (strict)"("XScale.Maximum"=600.0 ("X Scale.Range:Maximum"), "XScale.Minimum"=0.0 ("X Scale.Range:Minimum"), "YScale.Maximum"=100.0 ("Y Scale.Range:Maximum"), "YScale.Minimum"=0.0 ("Y Scale.Range:Minimum")) -> ()  [unwired: 2 in, 2 out]
          }
        }
      }
      frame "Compare Files" {
        # "Elapsed time\ncof\nstroke\nAir temp\nTemp\nHumidity"
        n2918 = case shown="True" "RSTV1 2" {
          frame False {
          }
          frame True {
            n2919 = property on="Humidity ( %RH )" class="XYGraph (strict)"("Y Scale.Display Format:Precision"=u8 0 ("Y Scale.Format & Precision:Precision")) -> ()  [unwired: 2 in, 2 out]
            n2920 = property on="Humidity ( %RH )" class="XYGraph (strict)"("X Scale.Range:Minimum"=0.0, "X Scale.Range:Maximum"=75.0, "Y Scale.Range:Minimum"=48.0, "Y Scale.Range:Maximum"=58.0) -> ()  [unwired: 2 in, 2 out]
          }
        }
        n2921 = case shown="True" "RST CP 2" {
          frame False {
          }
          frame True {
            n2922 = property on="XY Graph 13" class="XYGraph (strict)"("Y Scale.Display Format:Precision"=u8 0 ("Y Scale.Format & Precision:Precision")) -> ()  [unwired: 2 in, 2 out]
            n2923 = property on="XY Graph 13" class="XYGraph (strict)"("X Scale.Range:Minimum"=0.0, "X Scale.Range:Maximum"=75.0, "Y Scale.Range:Minimum"=0.0, "Y Scale.Range:Maximum"=100.0) -> ()  [unwired: 2 in, 2 out]
          }
        }
        n2924 = case shown="True" "RST CP" {
          frame False {
          }
          frame True {
            n2925 = property on="Sample Temperature ( °C )" class="XYGraph (strict)"("Y Scale.Display Format:Precision"=u8 2 ("Y Scale.Format & Precision:Precision")) -> ()  [unwired: 2 in, 2 out]
            n2926 = property on="Sample Temperature ( °C )" class="XYGraph (strict)"("X Scale.Range:Minimum"=0.0, "X Scale.Range:Maximum"=75.0, "Y Scale.Range:Minimum"=58.0, "Y Scale.Range:Maximum"=62.0) -> ()  [unwired: 2 in, 2 out]
          }
        }
        n2927 = case shown="True" "RSTV1 3" {
          frame False {
          }
          frame True {
            n2928 = property on="Air Temperature  ( °C )" class="XYGraph (strict)"("Y Scale.Display Format:Precision"=u8 2 ("Y Scale.Format & Precision:Precision")) -> ()  [unwired: 2 in, 2 out]
            n2929 = property on="Air Temperature  ( °C )" class="XYGraph (strict)"("X Scale.Range:Minimum"=0.0 ("Y Scale.Range:Minimum"), "X Scale.Range:Maximum"=75.0 ("Y Scale.Range:Maximum"), "Y Scale.Range:Minimum"=20.0 ("X Scale.Range:Minimum"), "Y Scale.Range:Maximum"=26.0 ("X Scale.Range:Maximum")) -> ()  [unwired: 2 in, 2 out]
          }
        }
        n2930 = case shown="True" "RSTV1 4" {
          frame False {
          }
          frame True {
            n2931 = property on="Stroke ( mm )" class="XYGraph (strict)"("Y Scale.Display Format:Precision"=u8 2 ("Y Scale.Format & Precision:Precision")) -> ()  [unwired: 2 in, 2 out]
            n2932 = property on="Stroke ( mm )" class="XYGraph (strict)"("X Scale.Range:Minimum"=0.0 ("Y Scale.Range:Maximum"), "X Scale.Range:Maximum"=75.0 ("X Scale.Range:Minimum"), "Y Scale.Range:Minimum"=0.98, "Y Scale.Range:Maximum"=1.02) -> ()  [unwired: 2 in, 2 out]
          }
        }
        n2933 = case shown="True" "rstv2" {
          frame False {
          }
          frame True {
            n2934 = property on="Coefficient Of Friction" class="XYGraph (strict)"("Y Scale.Display Format:Precision"=u8 3 ("Y Scale.Format & Precision:Precision")) -> ()  [unwired: 2 in, 2 out]
            n2935 = property on="Coefficient Of Friction" class="XYGraph (strict)"("X Scale.Range:Minimum"=0.0 ("Y Scale.Range:Maximum"), "X Scale.Range:Maximum"=75.0, "Y Scale.Range:Minimum"=0.0, "Y Scale.Range:Maximum"=1.0 ("X Scale.Range:Minimum")) -> ()  [unwired: 2 in, 2 out]
          }
        }
        n2936 = case shown="True" "RST CP 3" {
          frame False {
          }
          frame True {
            n2937 = property on="Air Temp ( °C ) vs Humidity ( % RH )" class="XYGraph (strict)"("X Scale.Range:Minimum"=18.0, "X Scale.Range:Maximum"=28.0 ("X Scale.Range:Minimum"), "Y Scale.Range:Minimum"=30.0 ("X Scale.Range:Minimum"), "Y Scale.Range:Maximum"=70.0 ("X Scale.Range:Minimum")) -> ()  [unwired: 2 in, 2 out]
          }
        }
        n2938 = case shown="True" "OPEN 1" {
          frame False {
          }
          frame True {
            (unwired) 0  # existing file
            w3665 = "Choose a datalog file to open"  # prompt
            n2939 = local write "OPEN 1"(FALSE ("OPEN 1")) -> ()
            n2940 = String To Path(string="C:\\LAB-IQ\\Data\\") -> (path=w3650:path)
            n2941 = File Dialog(6:"*.dgf" ("pattern"), 7:w3665, 11:w3650) -> (0:w3648:errorcluster, 3:w3656:path)  [unwired: 4 in, 2 out]
            n2942 = Unbundle(w3648) -> ()  [unwired: 3 out]
            n2943 = Strip Path(path=w3656) -> (name=w3655:string)  [unwired: 1 out]
            n2944 = Path To String(path=w3656) -> (string=w3651:string)
            "string1" <- w3651
            n2945 = Match Pattern(string=w3655, regular expression=".dgf") -> (before substring=→"String Control":string)  [unwired: 1 in, 3 out]
            n2946 = Match Pattern(string=w3651, regular expression=".dgf" ("substring (\"\")")) -> (before substring=w3661:string)  [unwired: 1 in, 3 out]
            n2947 = Concatenate Strings(w3661, ".duf" ("Substring")) -> (w3657:string)
            n2948 = String To Path(string=w3657) -> (path=w3662:path)
            n2949 = call <vilib>:"Read Characters From File.vi"("file path (dialog if empty)"=w3662, "start of read offset (chars.:0)"=60 ("start of read offset (chars.: 0)")) -> ("character string"=→"String Control 2":string)  [unwired: 4 in, 3 out]
          }
        }
        n2950 = case shown="True" "OPEN 2" {
          frame False {
          }
          frame True {
            (unwired) 0  # existing file
            w3683 = "Choose a datalog file to open"  # prompt
            n2951 = local write "OPEN 2"(FALSE ("OPEN 1")) -> ()
            n2952 = String To Path(string="C:\\LAB-IQ\\Data\\") -> (path=w3668:path)
            n2953 = File Dialog(6:"*.dgf" ("pattern"), 7:w3683, 11:w3668) -> (0:w3666:errorcluster, 3:w3674:path)  [unwired: 4 in, 2 out]
            n2954 = Unbundle(w3666) -> ()  [unwired: 3 out]
            n2955 = Strip Path(path=w3674) -> (name=w3672:string)  [unwired: 1 out]
            n2956 = Path To String(path=w3674) -> (string=w3669:string)
            "string1 2" <- w3669
            n2957 = Match Pattern(string=w3672, regular expression=".dgf") -> (before substring=→"String Control 3":string)  [unwired: 1 in, 3 out]
            n2958 = Match Pattern(string=w3669, regular expression=".dgf" ("substring (\"\")")) -> (before substring=w3680:string)  [unwired: 1 in, 3 out]
            n2959 = Concatenate Strings(w3680, ".duf" ("Substring")) -> (w3677:string)
            n2960 = String To Path(string=w3677) -> (path=w3675:path)
            n2961 = call <vilib>:"Read Characters From File.vi"("file path (dialog if empty)"=w3675, "start of read offset (chars.:0)"=60 ("start of read offset (chars.: 0)")) -> ("character string"=→"String Control 4":string)  [unwired: 4 in, 3 out]
          }
        }
        n2962 = case shown="True" "OPEN 3" {
          frame False {
          }
          frame True {
            (unwired) 0  # existing file
            w3701 = "Choose a datalog file to open"  # prompt
            n2963 = local write "OPEN 3"(FALSE ("OPEN 1")) -> ()
            n2964 = String To Path(string="C:\\LAB-IQ\\Data\\") -> (path=w3686:path)
            n2965 = File Dialog(6:"*.dgf" ("pattern"), 7:w3701, 11:w3686) -> (0:w3684:errorcluster, 3:w3692:path)  [unwired: 4 in, 2 out]
            n2966 = Unbundle(w3684) -> ()  [unwired: 3 out]
            n2967 = Strip Path(path=w3692) -> (name=w3690:string)  [unwired: 1 out]
            n2968 = Path To String(path=w3692) -> (string=w3687:string)
            "string1 3" <- w3687
            n2969 = Match Pattern(string=w3690, regular expression=".dgf") -> (before substring=→"String Control 5":string)  [unwired: 1 in, 3 out]
            n2970 = Match Pattern(string=w3687, regular expression=".dgf" ("substring (\"\")")) -> (before substring=w3697:string)  [unwired: 1 in, 3 out]
            n2971 = Concatenate Strings(w3697, ".duf" ("Substring")) -> (w3694:string)
            n2972 = String To Path(string=w3694) -> (path=w3698:path)
            n2973 = call <vilib>:"Read Characters From File.vi"("file path (dialog if empty)"=w3698, "start of read offset (chars.:0)"=60 ("start of read offset (chars.: 0)")) -> ("character string"=→"String Control 6":string)  [unwired: 4 in, 3 out]
          }
        }
        n2974 = case shown="True" "OPEN 4" {
          frame False {
          }
          frame True {
            (unwired) 0  # existing file
            w3719 = "Choose a datalog file to open"  # prompt
            n2975 = local write "OPEN 4"(FALSE ("OPEN 1")) -> ()
            n2976 = String To Path(string="C:\\LAB-IQ\\Data\\") -> (path=w3704:path)
            n2977 = File Dialog(6:"*.dgf" ("pattern"), 7:w3719, 11:w3704) -> (0:w3702:errorcluster, 3:w3710:path)  [unwired: 4 in, 2 out]
            n2978 = Unbundle(w3702) -> ()  [unwired: 3 out]
            n2979 = Strip Path(path=w3710) -> (name=w3708:string)  [unwired: 1 out]
            n2980 = Path To String(path=w3710) -> (string=w3705:string)
            "string1 4" <- w3705
            n2981 = Match Pattern(string=w3708, regular expression=".dgf") -> (before substring=→"String Control 7":string)  [unwired: 1 in, 3 out]
            n2982 = Match Pattern(string=w3705, regular expression=".dgf" ("substring (\"\")")) -> (before substring=w3715:string)  [unwired: 1 in, 3 out]
            n2983 = Concatenate Strings(w3715, ".duf" ("Substring")) -> (w3712:string)
            n2984 = String To Path(string=w3712) -> (path=w3716:path)
            n2985 = call <vilib>:"Read Characters From File.vi"("file path (dialog if empty)"=w3716, "start of read offset (chars.:0)"=60 ("start of read offset (chars.: 0)")) -> ("character string"=→"String Control 8":string)  [unwired: 4 in, 3 out]
          }
        }
      }
      frame "About" {
        # "Elapsed time\ncof\nstroke\nmean pos\nTemp\nHumidity"
        n2986 = disable-structure shown="Disabled" {
          frame Disabled {
            n2987 = case shown="True" "Export" {
              frame False {
              }
              frame True {
                w3741 = "                                      " ("string")
                w3743 = "\r"
                (unwired) i16 6 ("width (-)")
                w3820 = "\r"
                w3752 = "\r"
                n2988 = local write "Export"(FALSE ("Export")) -> ()
                n2989 = local read "String 29"() -> (w3789:string)
                n2990 = local read "String 34"() -> (w3777:string)
                n2991 = local read "String 35"() -> (w3772:string)
                n2992 = local read "String 37"() -> (w3768:string)
                n2993 = local read "String 36"() -> (w3765:string)
                n2994 = local read "String 38"() -> (w3762:string)
                n2995 = local read "String 39"() -> (w3759:string)
                n2996 = Match Pattern(string=w3789, regular expression=".dwm") -> (before substring=w3785:string)  [unwired: 1 in, 3 out]
                "before substring" <- w3785
                n2997 = local read "S 38"() -> (w3780:string)
                n2998 = local read "S 39"() -> (w3773:string)
                n2999 = local read "Temperature before test 2"() -> (w3809:dbl)
                n3000 = local read "Temperature after test 2"() -> (w3814:dbl)
                n3001 = local read "Humidity before test 2"() -> (w3795:dbl)
                n3002 = local read "Humidity after test 2"() -> (w3810:dbl)
                n3003 = local read "MWSD 2"() -> (w3806:dbl)
                n3004 = local read "WS1.4 2"() -> (w3822:dbl)
                n3005 = local read "HCF 2"() -> (w3818:dbl)
                n3006 = local read "AVP 2"() -> (w3807:dbl)
                n3007 = Concatenate Strings("1," ("string"), w3780) -> (w3779:string)
                n3008 = Concatenate Strings("2," ("string"), w3777) -> (w3776:string)
                n3009 = Concatenate Strings("3," ("string"), w3773) -> (w3775:string)
                n3010 = Concatenate Strings("4," ("string"), w3772) -> (w3771:string)
                n3011 = Concatenate Strings("5," ("string"), w3768) -> (w3769:string)
                n3012 = Concatenate Strings("6," ("string"), w3765) -> (w3766:string)
                n3013 = Concatenate Strings("7," ("string"), w3762) -> (w3763:string)
                n3014 = Concatenate Strings("8," ("string"), w3759) -> (w3760:string)
                n3015 = local read "Sample ID"() -> (w3827:string)
                n3016 = case shown="\"xlx\"" "Select File Type" {
                  tunnel: w3785 -> [w3830 w3832 w3834]
                  tunnel: [w3828 w3833 w3835] -> w3784
                  frame "xlx" {
                    n3017 = Concatenate Strings(w3830, ".xls" ("string")) -> (w3828:string)
                  }
                  frame "csv" {
                    n3018 = Concatenate Strings(w3832, ".csv" ("string")) -> (w3833:string)
                  }
                  frame "txt" {
                    n3019 = Concatenate Strings(w3834, ".txt" ("string")) -> (w3835:string)
                  }
                }
                n3020 = local read "Test Date"() -> (w3826:string)
                n3021 = local read "String 45"() -> (w3740:string)
                n3022 = local read "String 31"() -> (w3825:string)
                n3023 = local read "String 32"() -> (w3824:string)
                n3024 = local read "TITTLE"() -> (w3748:string)
                n3025 = Number To Fractional String(number=w3795, width (-)=i16 6, precision (6)=i16 2) -> (F-format string=w3794:string)  [unwired: 1 in]
                n3026 = Number To Fractional String(number=w3809, width (-)=i16 6, precision (6)=i16 2) -> (F-format string=w3815:string)  [unwired: 1 in]
                n3027 = Number To Fractional String(number=w3810, width (-)=i16 6, precision (6)=i16 2) -> (F-format string=w3808:string)  [unwired: 1 in]
                n3028 = Number To Fractional String(number=w3814, width (-)=i16 6, precision (6)=i16 2) -> (F-format string=w3813:string)  [unwired: 1 in]
                n3029 = Number To Fractional String(number=w3806, width (-)=i16 6, precision (6)=i16 2) -> (F-format string=w3804:string)  [unwired: 1 in]
                n3030 = Number To Fractional String(number=w3807, width (-)=i16 6, precision (6)=i16 2) -> (F-format string=w3805:string)  [unwired: 1 in]
                n3031 = Number To Fractional String(number=w3818, width (-)=i16 6, precision (6)=i16 2) -> (F-format string=w3819:string)  [unwired: 1 in]
                n3032 = Number To Fractional String(number=w3822, precision (6)=i16 2) -> (F-format string=w3823:string)  [unwired: 2 in]
                n3033 = local read "s.NO"() -> (w3742:string)
                n3034 = Concatenate Strings("=" ("string"), w3748) -> (w3747:string)
                n3035 = Concatenate Strings("S.No," ("string"), "                                       Parameters" ("string")) -> (w3753:string)
                n3036 = Concatenate Strings(w3820, w3779, w3794, w3820, w3776, w3815, w3820, w3775, w3808, w3820, w3771, w3813, w3820, w3769, w3804, w3820, w3766, w3805, w3820, w3763, w3819, w3820, w3760, w3823) -> (w3782:string)
